vi "GetScriptFromIni.vi"(8 "ErrorArray":errorcluster[](array[cluster]), 11 "PathtoIniFile":path=path "D:/Projects/Framework/Events/EventPlugins/C37EvtPlugin/C37EventPlugin.ini") -> (0 "ErrorArray":errorcluster[](array[cluster]), 2 "Script":string[](array[string]))   [LabVIEW 2014, in "Bus_class.lvlib" / "Bus.lvclass"]
uses:
  Bus.lvclass
  <vilib>/Utility/config.llb/NI_LVConfig.lvlib
  <userlib>/NIST/NISTErrorLib/NISTErrorLib.lvlib
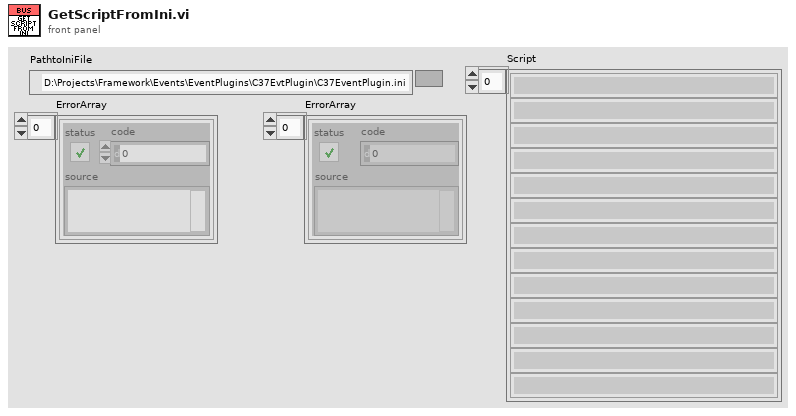
[diagram p1: front panel]
types:
  T1 = typedef "NI_LVConfig.lvlib/Config Data RefNum.ctl" = refnum<k1>
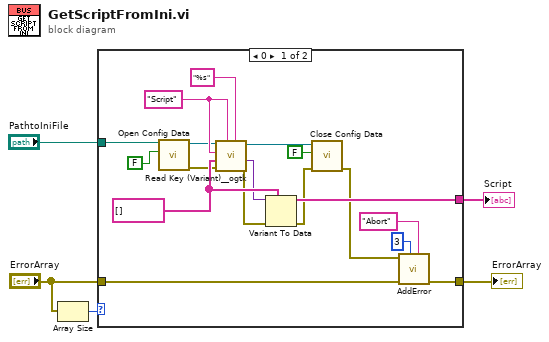
[diagram p0: block diagram]
diagram:
  n1 = Array Size(array="ErrorArray") -> (size(s)=w2:i32)
  n2 = case shown="0" w2 {
    tunnel: [w22 _] -> w5
    tunnel: "PathtoIniFile" -> [w11 _]
    tunnel: "ErrorArray" -> [w8 w24]
    tunnel: [w6 w24] -> w3
    frame 0 {
      w21 = string[] []
      w23 = "Script" ("section")
      n3 = call <vilib>:"Open Config Data.vi"("create file if necessary (T)"=FALSE, "configuration file path"=w11) -> ("error out"=w13:errorcluster, "refnum"=w14:T1)  [unwired: 7 in, 1 out]
      n4 = call <userlib>:"Read Key (Variant)__ogtk.vi"("format string (%;%f)"="%s", "section"=w23, "error in (no error)"=w13, "type"=w21, "key (optional)"=w23, "refnum"=w14) -> ("error out"=w18:errorcluster, "key-value"=w17:variant, "refnum out"=w15:T1)  [unwired: 2 in, 1 out]
      n5 = Variant To Data(error in=w18, type=w21, Variant=w17) -> (data=w22:string[], error out=w19:errorcluster)
      n6 = call <vilib>:"Close Config Data.vi"("error in (no error)"=w19, "write file if changed (T)"=FALSE, "refnum"=w15) -> ("error out"=w7:errorcluster)  [unwired: 7 in, 1 out]
      n7 = call <userlib>:"AddError.vi"("Severity"="Abort" ("String"), "Priority"=u8 3, "ErrorArray"=w8, "error in (no error)"=w7) -> ("ErrorArray"=w6:errorcluster[])  [unwired: 6 in, 1 out]
    }
    frame 1, Default {
    }
  }
  "Script" <- w5
  "ErrorArray" <- w3
